vi "XL320_Generate Serial String.vi"(0 "Motor ID":u8, 5 "Select Action":T1=3 items=["Ping"=1, "Read"=2, "Write"=3, "Registered Write"=4, "Action"=5, "Reset"=6, "Reboot"=8, "Status"=85, "Sync Read"=130, "Sync Write"=131, "Bulk Read"=146, "Bulk Write"=147], 7 "Address":u16, 9 "Parameters":string, 11 "Error in (no error)":errorcluster) -> (4 "Command to Serial":string, 15 "error out":errorcluster)   [LabVIEW 2017, in "Dynamixel XL320.lvlib"]
doc: "Generates a valid serial string that can be sent to the motor(s). This is a Low-Level VI that is used by other VIs."
uses:
  <instrlib>/Dynamixel XL320 (Drivers instrument)/Dynamixel XL320.lvlib
  <instrlib>/Dynamixel XL320 (Drivers instrument)/Public/Configure/XL320_Select_Action.ctl
panel:
  # "Ghislain REMY, IUT de Cachan, 2015 December 2015"
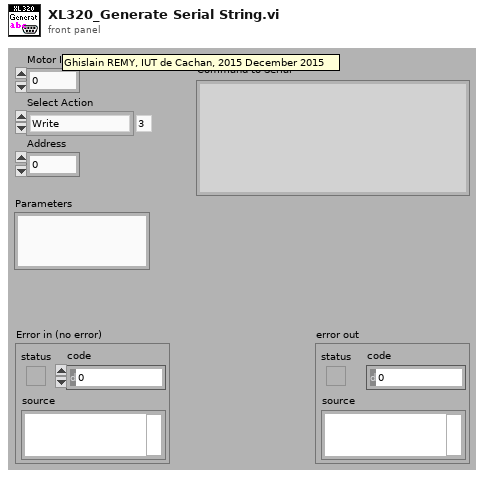
[diagram p1: front panel]
types:
  T1 = typedef "Dynamixel XL320.lvlib/XL320_Select_Action.ctl" = u8
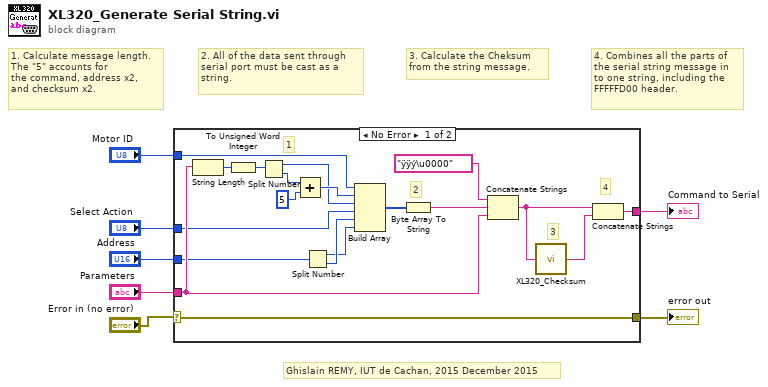
[diagram p0: block diagram]
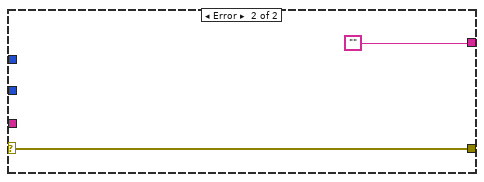
[diagram p2: hidden frame]
diagram:
  # "Ghislain REMY, IUT de Cachan, 2015 December 2015"
  # "3. Calculate the Cheksum \nfrom the string message."
  # "1. Calculate message length.\nThe \"5\" accounts for\nthe command, address x2,\nand checksum x2."
  # "2. All of the data sent through \nserial port must be cast as a \nstring."
  # "4. Combines all the parts of \nthe serial string message in \nto one string, including the \nFFFFFD00 header."
  n1 = case shown="No Error" "Error in (no error)" {
    selector: "Error in (no error)" -> [w23 w28]
    tunnel: "Address" -> [w14 _]
    tunnel: "Select Action" -> [w21 _]
    tunnel: "Motor ID" -> [w25 _]
    tunnel: [w18 ""] -> w5
    tunnel: [w23 w28] -> w4
    tunnel: "Parameters" -> [w22 _]
    frame No Error {
      # "4"
      # "3"
      # "2"
      # "1"
      n2 = String Length(string=w22) -> (length=w15:i32)
      n3 = To Unsigned Word Integer(number=w15) -> (unsigned 16bit integer=w13:u16)
      n4 = Split Number(x=w13) -> (hi(x)=w10:u8, lo(x)=w9:u8)
      n5 = Add(x=w9, y=u8 5) -> (x+y=w20:u8)
      n6 = Split Number(x=w14) -> (hi(x)=w11:u8, lo(x)=w12:u8)
      n7 = Build Array(w25, w20, w10, w21, w12, w11) -> (w19:T1[])
      n8 = Byte Array To String(unsigned byte array=w19) -> (string=w24:string)
      n9 = Concatenate Strings("ÿÿý\u0000", w24, w22) -> (w16:string)
      n10 = call <instrlib>:"XL320_Checksum.vi"("Input String"=w16) -> ("Checksum String"=w17:string)
      n11 = Concatenate Strings(w16, w17) -> (w18:string)
    }
    frame Error {
    }
  }
  "Command to Serial" <- w5
  "error out" <- w4
